vi "将数组行倒序.vi"(9 "新数据数组":string[](array[string]), 10 "原有数组":string[][](array[string])) -> (1 "倒序后的数组":string[][](array[string]))   [LabVIEW 2017]
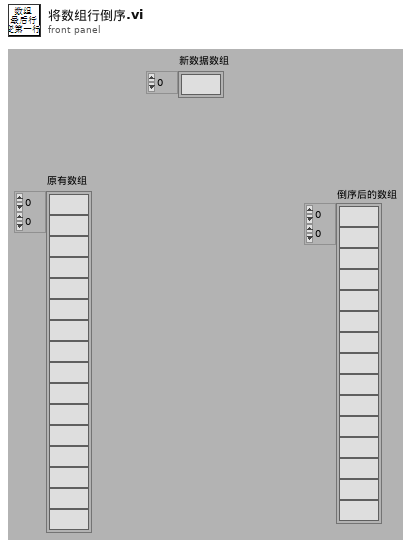
[diagram p1: front panel]
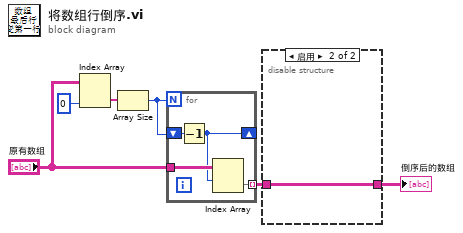
[diagram p0: block diagram]
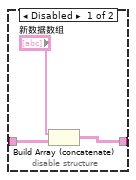
[diagram p2: hidden frame]
diagram:
  n1 = Index Array(array="原有数组", index (col)=0 ("禁用的索引 (列)")) -> (element=w3:string[])  [unwired: 1 in]
  n2 = Array Size(array=w3) -> (size(s)=w1:i32)
  n3 = for {
    N: w1 -> [_]
    tunnel: "原有数组" -> [w10]
    tunnel: [w9] -> w2 mode=indexing
    shift-right: [w7] -> _
    shift-left: w1 -> [w8]
    n4 = Decrement(x=w8) -> (x-1=w7:i32)
    n5 = Index Array(array=w10, index (row)=w7) -> (element=w9:string[])  [unwired: 1 in]
  }
  n6 = disable-structure shown="启用" {
    disable-tunnel: [w12 w14] -> w6
    disable-tunnel: w2 -> [w11 w14]
    frame Disabled {
      n7 = Build Array (concatenate)("新数据数组", w11) -> (w12:string[][])
    }
    frame Enabled {
    }
  }
  "倒序后的数组" <- w6
